vi "MicroPLSavePanel.vi"(8 "error in":errorcluster) -> (0 "error out":errorcluster, 3 "Chaîne":string)   [LabVIEW 2019, in "PhotoLum.lvclass"]
uses:
  PhotoLum.lvclass
panel:
  in  "Objectif":u16(ring) items=["5x", "10x", "20x", "40x", "60x"]
  in  "NDFilter2":u16(ring) caption="Filtre ND 2" items=["Vide", "0.3 OD", "1.0 OD", "2.0 OD", "3.0 OD", "4.0 OD"]
  in  "NDFilter1":u16(ring) caption="Filtre ND 1" items=["Vide", "0.2 OD", "0.4 OD", "0.5 OD", "0.6 OD", "4.0 OD"]
  in  "SlitHeightOut":u16(ring) caption="Hauteur fente de sortie" items=["15 mm", "1 mm"]
  in  "OtherMat":string caption="Matériaux (autres)"
  in  "Matériaux":u16(ring) items=["AlGaAs", "AlP", "GaAs", "GaN", "Ge", "InP", "Si", "Diamond", "SiGe", "Autres"]
  in  "unit":u16(ring) caption="Unités\nPre-amp." items=["mA/V", "µA/V", "nA/V", "pA/V"]
  in  "Facteur":u16(ring) caption="Facteur Pre-amp." items=["1", "2", "5", "10", "20", "50", "100", "200", "500"]
  in  "Preamp":u16(ring) caption="Pre-amplificateur" items=["Aucun", "SR570 Current Preamp", "SR560 Voltage Preamp"]
  in  "PLaser":dbl=250.0 caption="Puissance(mW)" min=0.0 step=0.1 format="%#.1f"
  in  "Temp":dbl=293.0 caption="Température(K)" min=0.0 step=0.1 format="%#.1f"
  in  "Annuler":bool
  in  "Save":bool
  in  "Autres":string
  in  "Filtre":u16(ring)=5 caption="Filtre Entrée" items=["Aucun", "UV 365nm", "Mauve", "Jaune 495nm", "Vert", "Orange 550nm", "Rouge 665nm", "Rouge 850nm", "SI"]
  in  "LN Cooled":bool
  in  "Échantillon":string
  in  "Excitation":u16(ring)=1 caption="Source d'excitation" items=["Diode 266nm", "Diode 532nm"]
  in  "Détecteur":u16(ring)=1 items=["Symphony Camera", "Photon Counter R2949", "PM Hamamatsu R9268", "Détecteur Ge EG&G", "Détecteur Si EG&G", "Détecteur InAs EG&G", "Détecteur InSb EG&G"]
  in  "SlitHeight":u16(ring) caption="Hauteur fente d'entrée" items=["15 mm", "1 mm"]
  # "Paramètres du balayage"
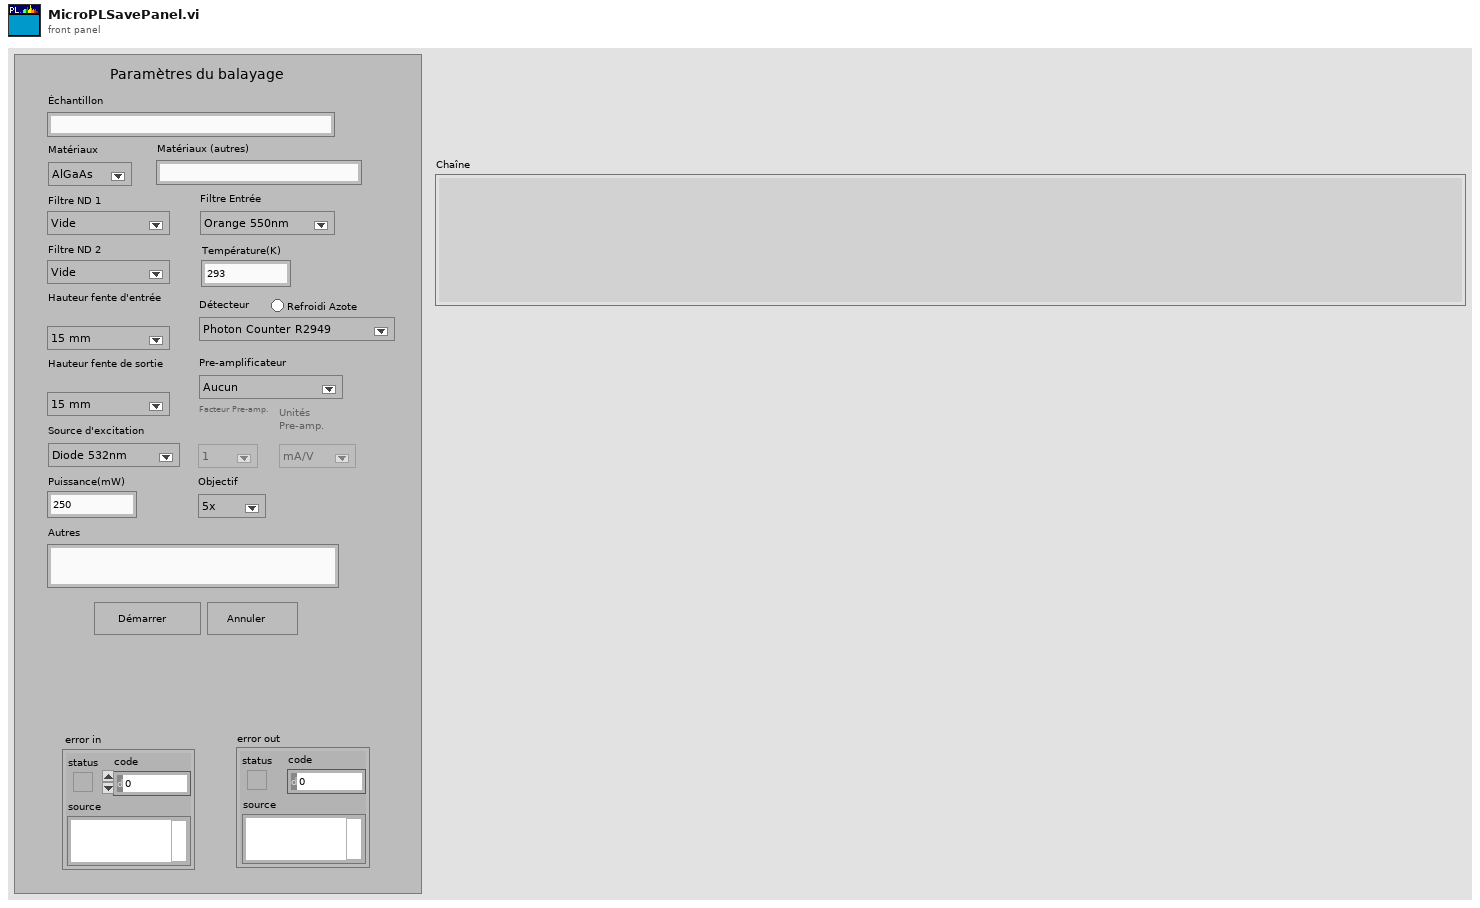
[diagram p1: front panel]
types:
  T1 = enum8{"Enabled", "Disabled", "Disabled and Grayed Out"}
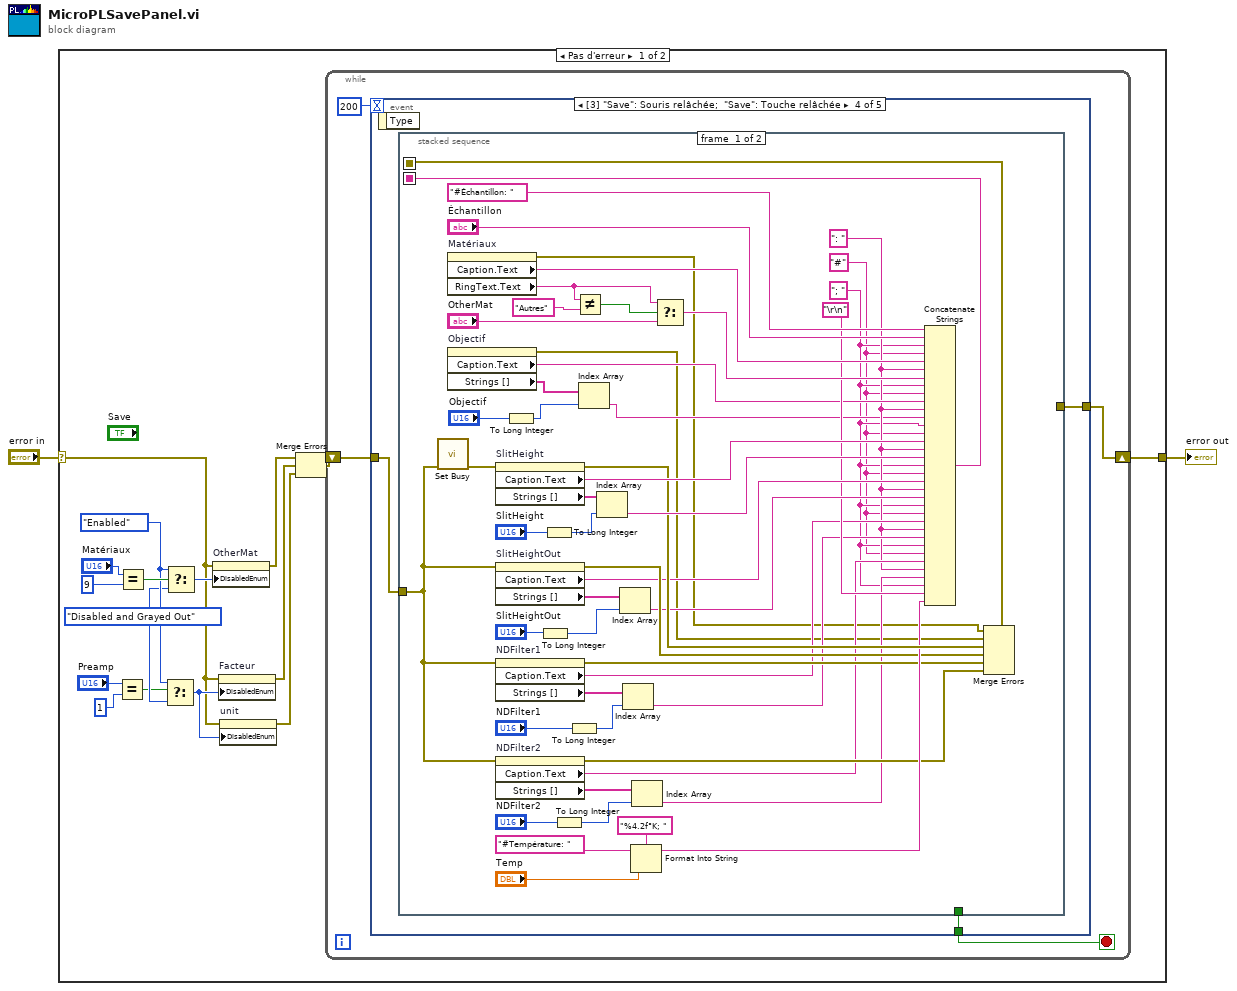
[diagram p0: block diagram]
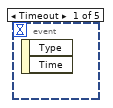
[diagram p2: hidden frame]
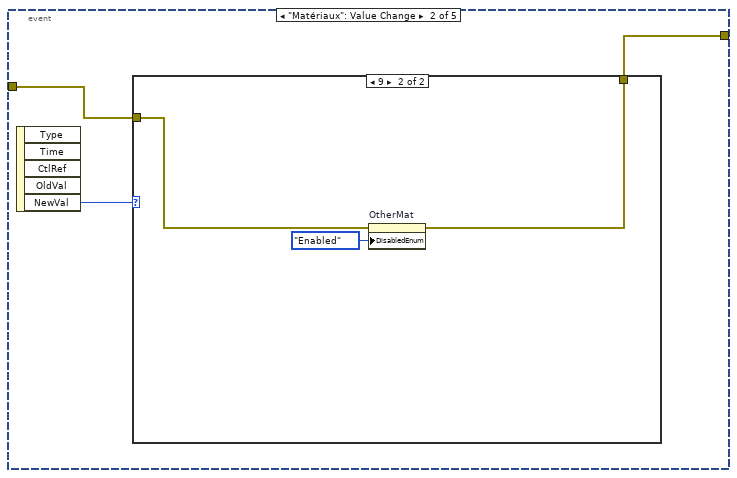
[diagram p3: hidden frame]
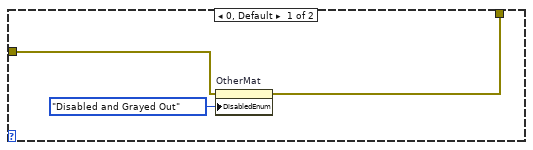
[diagram p4: hidden frame]
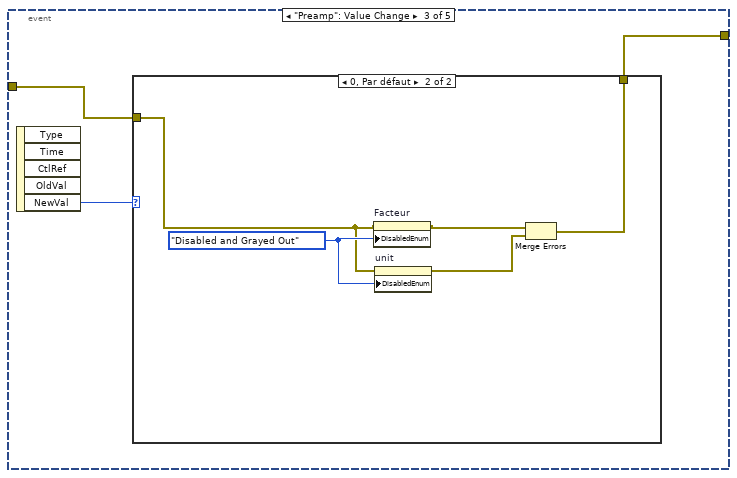
[diagram p5: hidden frame]
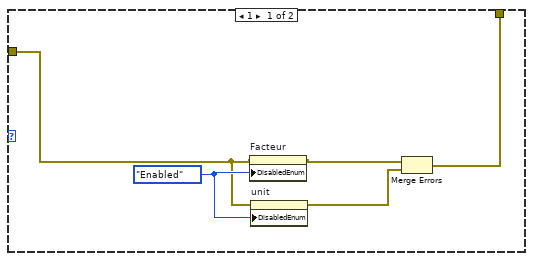
[diagram p6: hidden frame]
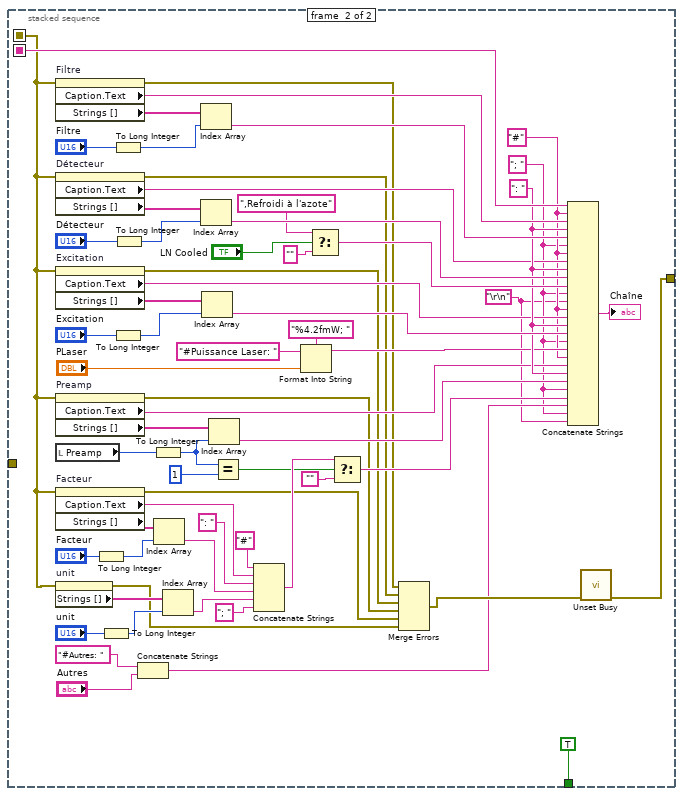
[diagram p7: hidden frame]
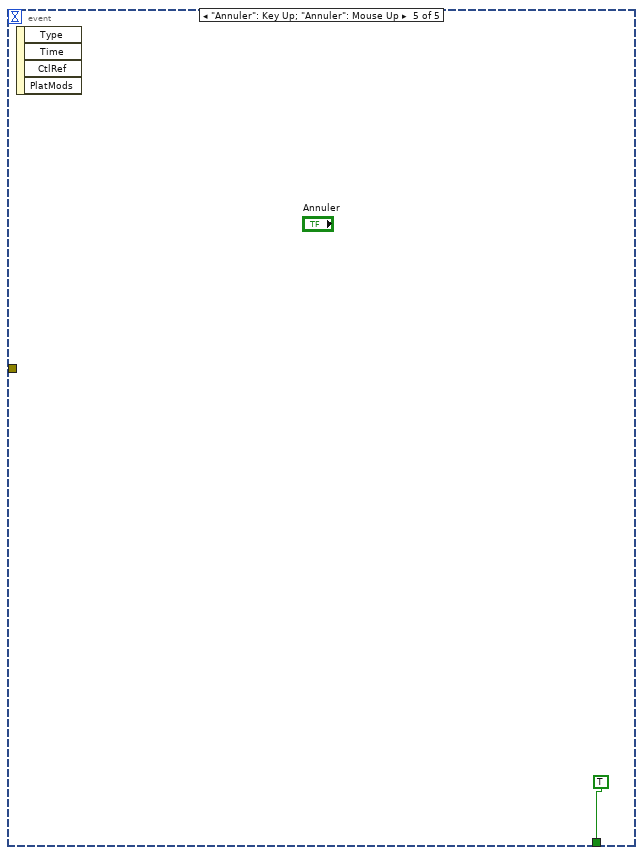
[diagram p8: hidden frame]
diagram:
  n1 = case shown="Pas d'erreur" "error in" {
    selector: "error in" -> [w6 w164]
    tunnel: [w18 w164] -> w2
    frame No Error {
      w9 = T1."Disabled and Grayed Out" ("Désactivé")
      w10 = T1."Enabled" ("Désactivé")
      n2 = Equal?(x="Preamp", y=1) -> (x = y?=w8:bool)
      n3 = Equal?(x="Matériaux", y=u16 9) -> (x = y?=w15:bool)
      n4 = Select(t=w10, s=w8, f=w9) -> (s? t:f=w7:T1)
      n5 = Select(t=w10, s=w15, f=w9) -> (s? t:f=w14:T1)
      n6 = property on="OtherMat" class="Ch"(error in=w6, "DisabledEnum"=w14) -> (error out=w13:errorcluster)  [unwired: 1 in, 1 out]
      n7 = property on="Facteur" class="MDér (strict)"(error in=w6, "DisabledEnum"=w7) -> (error out=w4:errorcluster)  [unwired: 1 in, 1 out]
      n8 = property on="unit" class="MDér (strict)"(error in=w6, "DisabledEnum"=w7) -> (error out=w3:errorcluster)  [unwired: 1 in, 1 out]
      n9 = Merge Errors(w13, w4, w3) -> (w5:errorcluster)
      n10 = while {
        shift-right: [w19] -> w18
        shift-left: w5 -> [w20]
        stop <- w21 stop-if-true
        n11 = event shown="[3] \"Save\": Souris relâchée;  \"Save\": Touche relâchée" {
          selector: _ -> [_ _ _ _ _]
          dyn-events: _ -> [_ _ _ _ _]
          timeout: 200 -> [_ _ _ _ _]
          tunnel: [_ _ _ w47 TRUE] -> w21
          tunnel: w20 -> [_ w24 w33 w46 _]
          tunnel: [_ w23 w32 w45 _] -> w19
          event Timeout {
            n12 = event-data() -> ()  [unwired: 1 in, 2 out]
          }
          event "Matériaux": Value Change {
            n13 = event-data() -> ("NewVal"=w25:u16)  [unwired: 1 in, 4 out]
            n14 = case shown="9" w25 {
              tunnel: w24 -> [w27 w30]
              tunnel: [w26 w29] -> w23
              frame 0, Default {
                n15 = property on="OtherMat" class="Ch"(error in=w27, "DisabledEnum"=T1."Disabled and Grayed Out" ("Désactivé")) -> (error out=w26:errorcluster)  [unwired: 1 in, 1 out]
              }
              frame 9 {
                n16 = property on="OtherMat" class="Ch"(error in=w30, "DisabledEnum"=T1."Enabled" ("Désactivé")) -> (error out=w29:errorcluster)  [unwired: 1 in, 1 out]
              }
            }
          }
          event "Preamp": Value Change {
            n17 = event-data() -> ("NewVal"=w34:u16)  [unwired: 1 in, 4 out]
            n18 = case shown="0, Par défaut" w34 {
              tunnel: w33 -> [w37 w42]
              tunnel: [w36 w41] -> w32
              frame 1 {
                w38 = T1."Enabled" ("Désactivé")
                n19 = property on="Facteur" class="MDér (strict)"(error in=w37, "DisabledEnum"=w38) -> (error out=w39:errorcluster)  [unwired: 1 in, 1 out]
                n20 = property on="unit" class="MDér (strict)"(error in=w37, "DisabledEnum"=w38) -> (error out=w35:errorcluster)  [unwired: 1 in, 1 out]
                n21 = Merge Errors(w39, w35) -> (w36:errorcluster)
              }
              frame 0, Default {
                w43 = T1."Disabled and Grayed Out" ("Désactivé")
                n22 = property on="Facteur" class="MDér (strict)"(error in=w42, "DisabledEnum"=w43) -> (error out=w44:errorcluster)  [unwired: 1 in, 1 out]
                n23 = property on="unit" class="MDér (strict)"(error in=w42, "DisabledEnum"=w43) -> (error out=w40:errorcluster)  [unwired: 1 in, 1 out]
                n24 = Merge Errors(w44, w40) -> (w41:errorcluster)
              }
            }
          }
          event "Save": Mouse Up; "Save": Key Up {
            n25 = event-data() -> ()  [unwired: 1 in, 1 out]
            n26 = stacked-sequence {
              seq-local: [w87 _] -> [_ w145]
              seq-local: [w79 _] -> [_ w107]
              tunnel: [_ TRUE] -> w47
              tunnel: w46 -> [w63 _]
              tunnel: [_ w105] -> w45
              frame #0 {
                w48 = "#" ("string")
                w53 = ": " ("string")
                w49 = "; " ("chaîne")
                n27 = call <vilib>:"Set Busy.vi"("error in (no error)"=w63) -> ("error out"=w88:errorcluster)  [unwired: 9 in, 1 out]
                n28 = property on="Matériaux" class="MDér (strict)"() -> (error out=w51:errorcluster, "Caption.Text"=w75:string, "RingText.Text"=w72:string)  [unwired: 2 in, 1 out]
                n29 = property on="Objectif" class="MDér (strict)"() -> (error out=w50:errorcluster, "Caption.Text"=w54:string, "Strings []"=w56:string[])  [unwired: 2 in, 1 out]
                n30 = property on="SlitHeight" class="MDér (strict)"(error in=w88) -> (error out=w86:errorcluster, "Caption.Text"=w93:string, "Strings []"=w96:string[])  [unwired: 1 in, 1 out]
                n31 = property on="SlitHeightOut" class="MDér (strict)"(error in=w63) -> (error out=w78:errorcluster, "Caption.Text"=w77:string, "Strings []"=w82:string[])  [unwired: 1 in, 1 out]
                n32 = property on="NDFilter1" class="MDér (strict)"(error in=w63) -> (error out=w65:errorcluster, "Caption.Text"=w61:string, "Strings []"=w70:string[])  [unwired: 1 in, 1 out]
                n33 = property on="NDFilter2" class="MDér (strict)"(error in=w63) -> (error out=w64:errorcluster, "Caption.Text"=w59:string, "Strings []"=w69:string[])  [unwired: 1 in, 1 out]
                n34 = To Long Integer(number="Objectif") -> (32bit integer=w55:i32)
                n35 = To Long Integer(number="SlitHeightOut") -> (32bit integer=w81:i32)
                n36 = To Long Integer(number="SlitHeight") -> (32bit integer=w95:i32)
                n37 = To Long Integer(number="NDFilter2") -> (32bit integer=w68:i32)
                n38 = To Long Integer(number="NDFilter1") -> (32bit integer=w71:i32)
                n39 = Not Equal?(x=w72, y="Autres") -> (x != y?=w73:bool)
                n40 = Index Array(array=w56, index=w55) -> (element=w52:string)
                n41 = Index Array(array=w96, index=w95) -> (element=w92:string)
                n42 = Index Array(array=w82, index=w81) -> (element=w76:string)
                n43 = Index Array(array=w70, index=w71) -> (element=w60:string)
                n44 = Format Into String(format string="%4.2f°K; " ("chaîne de format"), initial string="#Température: " ("string"), "Temp") -> (resulting string=w80:string)  [unwired: 1 in, 1 out]
                n45 = Index Array(array=w69, index=w68) -> (element=w58:string)
                n46 = Select(t=w72, s=w73, f="OtherMat") -> (s? t:f=w84:string)
                n47 = Concatenate Strings("#Échantillon: " ("chaîne"), "Échantillon", w49, w48, w75, w53, w84, w49, w48, w54, w53, w52, w49, w48, w93, w53, w92, w49, w48, w77, w53, w76, w49, w48, w61, w53, w60, w49, w48, w59, w53, w58, w49, "\r\n", w80) -> (w87:string)
                n48 = Merge Errors(w51, w50, w86, w78, w65, w64) -> (w79:errorcluster)
              }
              frame #1 {
                w114 = "#" ("chaîne")
                w100 = "\r\n"
                w101 = "; " ("chaîne")
                w143 = ": " ("chaîne")
                n49 = property on="Filtre" class="MDér (strict)"(error in=w107) -> (error out=w113:errorcluster, "Caption.Text"=w153:string, "Strings []"=w162:string[])  [unwired: 1 in, 1 out]
                n50 = property on="Détecteur" class="MDér (strict)"(error in=w107) -> (error out=w112:errorcluster, "Caption.Text"=w120:string, "Strings []"=w158:string[])  [unwired: 1 in, 1 out]
                n51 = property on="Excitation" class="MDér (strict)"(error in=w107) -> (error out=w111:errorcluster, "Caption.Text"=w117:string, "Strings []"=w155:string[])  [unwired: 1 in, 1 out]
                n52 = property on="Preamp" class="MDér (strict)"(error in=w107) -> (error out=w110:errorcluster, "Caption.Text"=w123:string, "Strings []"=w144:string[])  [unwired: 1 in, 1 out]
                n53 = local read "Preamp"() -> (w99:u16)
                n54 = property on="Facteur" class="MDér (strict)"(error in=w107) -> (error out=w109:errorcluster, "Caption.Text"=w127:string, "Strings []"=w134:string[])  [unwired: 1 in, 1 out]
                n55 = property on="unit" class="MDér (strict)"(error in=w107) -> (error out=w108:errorcluster, "Strings []"=w133:string[])  [unwired: 1 in, 1 out]
                n56 = To Long Integer(number="Facteur") -> (32bit integer=w130:i32)
                n57 = To Long Integer(number="unit") -> (32bit integer=w129:i32)
                n58 = To Long Integer(number="Filtre") -> (32bit integer=w160:i32)
                n59 = To Long Integer(number="Excitation") -> (32bit integer=w156:i32)
                n60 = To Long Integer(number="Détecteur") -> (32bit integer=w159:i32)
                n61 = Concatenate Strings("#Autres: " ("chaîne"), "Autres") -> (w102:string)
                n62 = To Long Integer(number=w99) -> (32bit integer=w138:i32)
                n63 = Index Array(array=w134, index=w130) -> (element=w125:string)
                n64 = Index Array(array=w133, index=w129) -> (element=w128:string)
                n65 = Index Array(array=w162, index=w160) -> (element=w152:string)
                n66 = Index Array(array=w158, index=w159) -> (element=w151:string)
                n67 = Index Array(array=w155, index=w156) -> (element=w150:string)
                n68 = Index Array(array=w144, index=w138) -> (element=w142:string)
                n69 = Equal?(x=w138, y=1) -> (x = y?=w121:bool)
                n70 = Concatenate Strings("#" ("chaîne"), w127, ": " ("chaîne"), w125, w128, "; " ("chaîne")) -> (w122:string)
                n71 = Format Into String(format string="%4.2fmW; " ("chaîne de format"), initial string="#Puissance Laser: " ("string"), "PLaser") -> (resulting string=w139:string)  [unwired: 1 in, 1 out]
                n72 = Select(t=",Refroidi à l'azote" ("chaîne"), s="LN Cooled", f="" ("chaîne")) -> (s? t:f=w146:string)
                n73 = Select(t=w122, s=w121, f="") -> (s? t:f=w135:string)
                n74 = Merge Errors(w113, w112, w111, w110, w109, w108) -> (w106:errorcluster)
                n75 = Concatenate Strings(w145, w114, w153, w143, w152, w101, w114, w120, w143, w151, w146, w101, w100, w114, w117, w143, w150, w101, w139, w114, w123, w143, w142, w101, w135, w102, w101, w100) -> (→"Chaîne":string)
                n76 = call <vilib>:"Unset Busy.vi"("error in (no error)"=w106) -> ("error out"=w105:errorcluster)  [unwired: 10 in]
              }
            }
          }
          event "Annuler": Key Up; "Annuler": Mouse Up {
            n77 = event-data() -> ()  [unwired: 1 in, 4 out]
          }
        }
      }
    }
    frame Error {
    }
  }
  "error out" <- w2
